vi "q4 flat sequence.vi"() -> ()   [LabVIEW 2018]
panel:
  out "Y":dbl
  in  "C":dbl
  in  "B":dbl
  in  "A":dbl
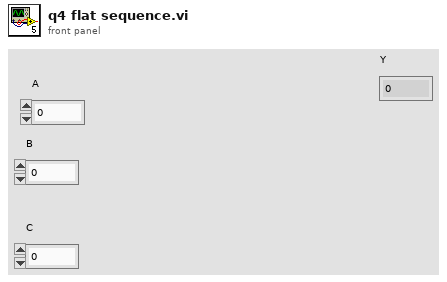
[diagram p1: front panel]
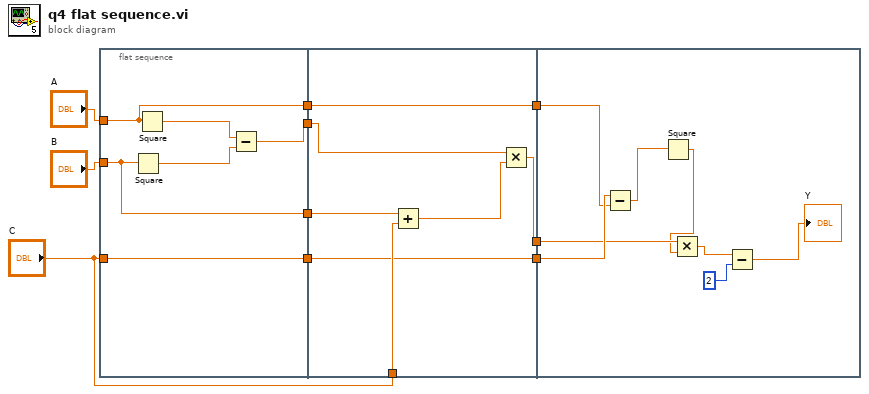
[diagram p0: block diagram]
diagram:
  n1 = flat-sequence {
    tunnel: "A" -> [w11]
    tunnel: "B" -> [w13]
    tunnel: [w14] -> w8
    tunnel: [w13] -> w7
    tunnel: "C" -> [w12]
    tunnel: [w12] -> w4
    tunnel: [w11] -> w2
    tunnel: w8 -> [w21]
    tunnel: w7 -> [w23]
    tunnel: "C" -> [w22]
    tunnel: [w19] -> w5
    tunnel: w4 -> [w19]
    tunnel: [w18] -> w3
    tunnel: w2 -> [w18]
    tunnel: [w17] -> w1
    tunnel: w5 -> [w31]
    tunnel: w3 -> [w30]
    tunnel: w1 -> [w28]
    frame #0 {
      n2 = Square(x=w13) -> (x^2=w15:dbl)
      n3 = Square(x=w11) -> (x^2=w16:dbl)
      n4 = Subtract(x=w16, y=w15) -> (x-y=w14:dbl)
    }
    frame #1 {
      n5 = Add(x=w23, y=w22) -> (x+y=w20:dbl)
      n6 = Multiply(x=w21, y=w20) -> (x*y=w17:dbl)
    }
    frame #2 {
      n7 = Subtract(x=w31, y=w30) -> (x-y=w29:dbl)
      n8 = Square(x=w29) -> (x^2=w27:dbl)
      n9 = Multiply(x=w28, y=w27) -> (x*y=w26:dbl)
      n10 = Subtract(x=w26, y=2) -> (x-y=→"Y":dbl)
    }
  }
